vi "Config Waitfor.vi"(8 "error in":errorcluster, 9 "Trigger Mode (Buffer)":u16(ring) items=["Buffer", "Error"], 10 "Sample Delay (0)":dbl min=0.0 max=99999999.8 step=0.01 format="%#_10g", 11 "VISA resource name":refnum<visa-resource-name>) -> (0 "error out":errorcluster, 3 "VISA resource name out":refnum<visa-resource-name>)   [LabVIEW 2017, in "Andeen-Hagerling 2700.lvlib"]
doc: "This VI specifies a time delay that automatically occurs following each change in the Sample (sample number) parameter. This provides a settling time for sample switch relays to stabilize after being switched. It also determines what happens to external trigger pulses that arrive when no command has been executed to receive them. This command allows such pulses to be buffered or to report an error. Execution of this command clears the trigger buffer."
uses:
  Andeen-Hagerling 2700.lvlib
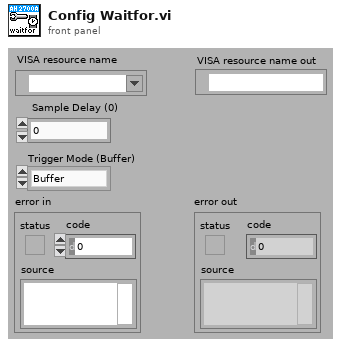
[diagram p1: front panel]
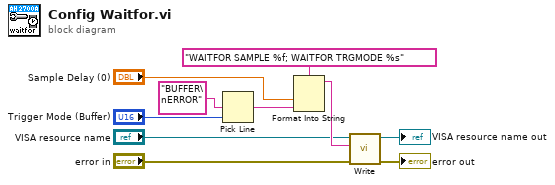
[diagram p0: block diagram]
diagram:
  n1 = Pick Line(multi-line string="BUFFER\nERROR", line index="Trigger Mode (Buffer)") -> (output string=w7:string)  [unwired: 1 in]
  n2 = Format Into String(format string="WAITFOR SAMPLE %f; WAITFOR TRGMODE %s", "Sample Delay (0)", w7) -> (resulting string=w5:string)  [unwired: 2 in, 1 out]
  n3 = call "Write.vi"("error in"="error in", "command"=w5, "VISA resource name"="VISA resource name") -> ("error out"=→"error out":errorcluster, "VISA resource name out"=→"VISA resource name out":refnum<visa-resource-name>)  [unwired: 7 in]
